vi "Goal Steer.vi"(8 "Reinit?":bool, 10 "Manual Steer":dbl) -> (2 "Steering Out":dbl)   [LabVIEW 2013]
uses:
  Common Code/Change Detect Boolean.vi
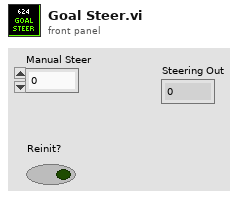
[diagram p1: front panel]
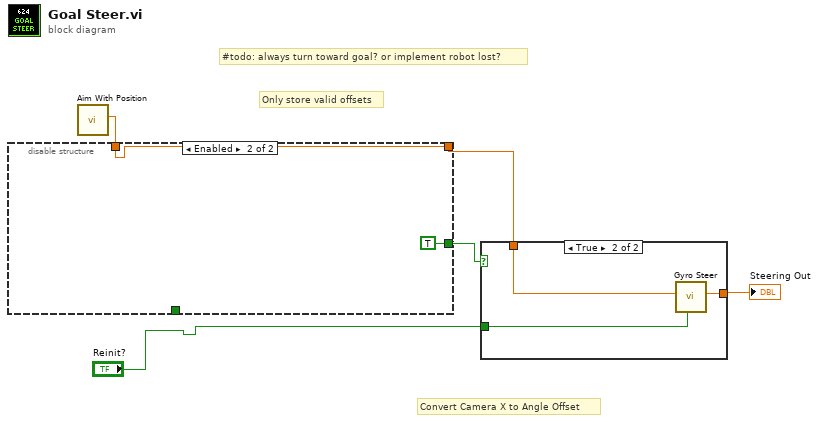
[diagram p0: block diagram]
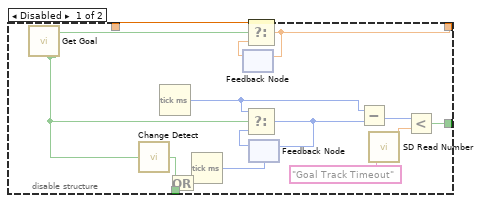
[diagram p2: hidden frame]
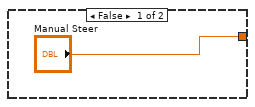
[diagram p3: hidden frame]
diagram:
  # "#todo: always turn toward goal? or implement robot lost?"
  # "Only store valid offsets"
  # "Convert Camera X to Angle Offset"
  n1 = call "Aim With Position.vi"() -> ("Target Gyro Angle"=w2:dbl)  [unwired: 9 in, 2 out]
  n2 = disable-structure shown="Enabled" {
    disable-tunnel: [w18 TRUE] -> w5
    disable-tunnel: [w13 _] -> _
    disable-tunnel: [w9 w20] -> w3
    disable-tunnel: w2 -> [w6 w20]
    frame Disabled {
      n3 = call "Get Goal.vi"() -> ("Goal Found?"=w7:bool)  [unwired: 8 in, 7 out]
      n4 = call-poly "Change Detect.vi"("In"=w7) -> ("Changed?"=w13:bool)
      n5 = Tick Count (ms)() -> (millisecond timer value=w12:u32)
      n6 = Or() -> ()  [unwired: 2 in, 1 out]
      n7 = Tick Count (ms)() -> (millisecond timer value=w15:u32)
      n8 = feedback #1() -> (w8:dbl)  [unwired: 1 in]
      n9 = Select(t=w6, s=w7, f=w8) -> (s? t:f=w9:dbl)
      n10 = feedback-in #1(w9) -> ()
      n11 = feedback #2(w15) -> (w11:u32)
      n12 = Select(t=w12, s=w7, f=w11) -> (s? t:f=w10:u32)
      n13 = feedback-in #2(w10) -> ()
      n14 = Subtract(x=w12, y=w10) -> (x-y=w16:u32)
      n15 = call <vilib>:"SD Read Number.vi"("Name"="Goal Track Timeout") -> ("Numeric"=w17:dbl)  [unwired: 8 in, 2 out]
      n16 = Less?(x=w16, y=w17) -> (x < y?=w18:bool)
    }
    frame Enabled {
    }
  }
  n17 = case shown="True" w5 {
    tunnel: "Reinit?" -> [_ w24]
    tunnel: ["Manual Steer" w23] -> w4
    tunnel: w3 -> [_ w22]
    frame False {
    }
    frame True {
      n18 = call "Gyro Steer.vi"("reinitialize? (F)"=w24, "Target Angle"=w22) -> ("Steering Out"=w23:dbl)  [unwired: 8 in, 1 out]
    }
  }
  "Steering Out" <- w4
